vi "Test_sqlite3CreateDatabaseAndATableWorks_NoError.vi"(8 "error in (no error)":errorcluster, 11 "TestCase in":refnum<class "Test sqlite3.lvclass">) -> (0 "error out":errorcluster, 3 "TestCase out":refnum<class "Test sqlite3.lvclass">)   [LabVIEW 2020, in "Test sqlite3.lvclass"]
uses:
  Test sqlite3.lvclass
  <vilib>/Utility/sysdir.llb/System Directory Type.ctl
  externals/sqlite3/Source/sqlite3.lvclass/sqlite3.ctl
  45a547b6-e4c0-49d6-ab78-a1d3563bf804.vi
  <vilib>/Utility/error.llb/Error Cluster From Error Code.vi
  externals/sqlite3/Source/sqlite3.lvclass
  <vilib>/addons/_JKI Toolkits/VI Tester/TestCase.llb/TestCase.lvclass
  externals/database-interface/IDatabase/IDatabase/IDatabase.lvclass
  C:/Program Files/National Instruments/LabVIEW 2020/vi.lib/addons/_JKI Toolkits/VI Tester/TestCase.llb/TestCase.lvclass
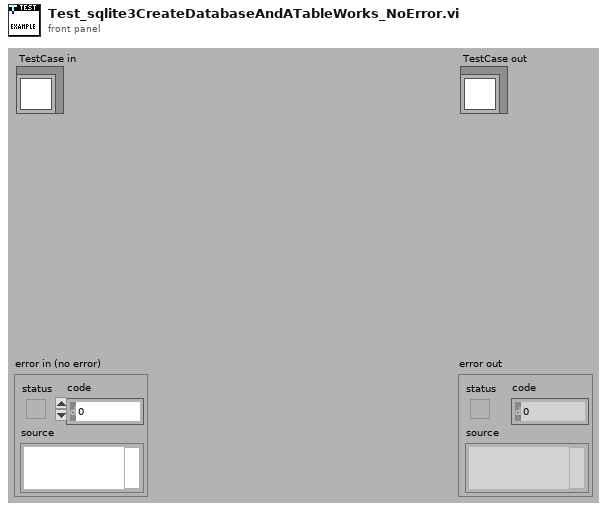
[diagram p1: front panel]
types:
  T1 = typedef "System Directory Type.ctl" = i32
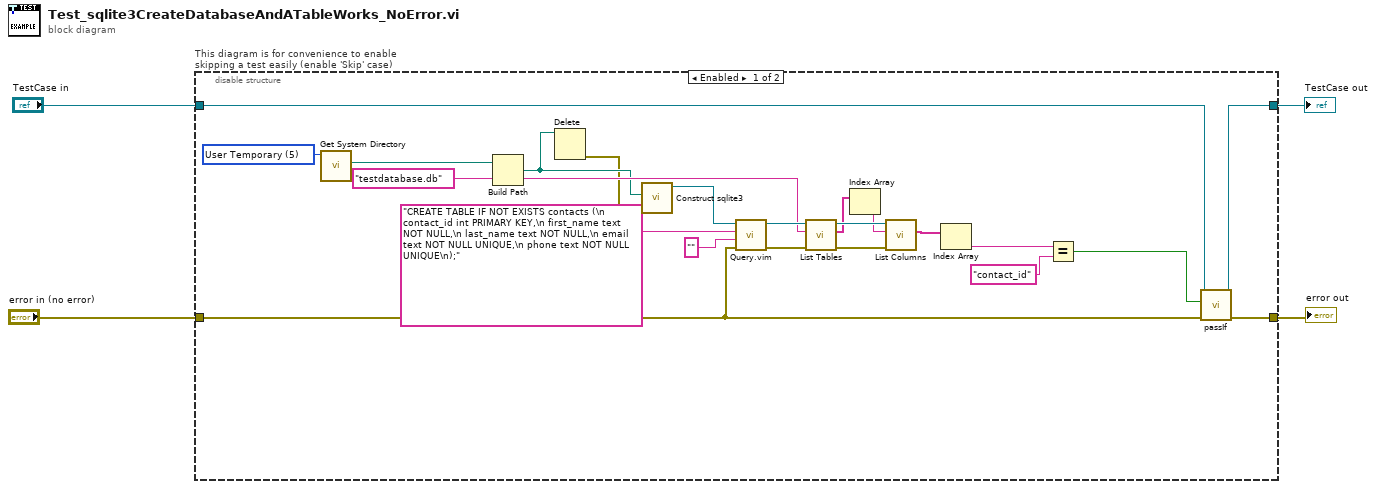
[diagram p0: block diagram]
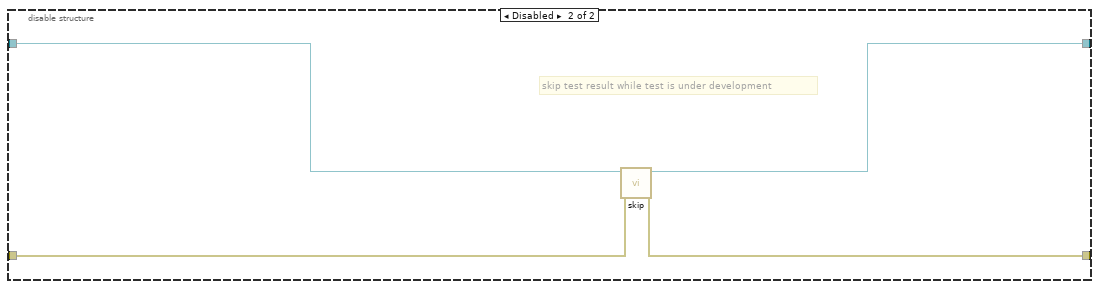
[diagram p2: hidden frame]
diagram:
  n1 = disable-structure "This diagram is for convenience to enable skipping a test easily (enable 'Skip' case)" shown="Enabled" {
    disable-tunnel: "TestCase in" -> [w24 w30]
    disable-tunnel: [w26 w28] -> w1
    disable-tunnel: [w25 w29] -> w3
    disable-tunnel: "error in (no error)" -> [w14 w27]
    frame Enabled {
      w20 = T1 5 items=["User Home"=0, "User Desktop"=1, "User Documents"=2, "User Application Data"=3, "User Preferences"=4, "User Temporary"=5, "Public Documents"=6, "Public Application Data"=7, "Public Preferences"=8, "Public Cache"=13, "System Core Libraries"=9, "System Installed Libraries"=10, "Application Files"=11, "Boot Volume Root"=12] ("system directory type")
      w13 = "testdatabase.db" ("name or relative path")
      n2 = call <vilib>:"Get System Directory.vi"("system directory type"=w20) -> ("system directory"=w19:path)  [unwired: 10 in]
      n3 = Build Path(base path=w19, name or relative path=w13) -> (appended path=w6:path)
      n4 = Delete(path (use dialog)=w6) -> (error out=w5:errorcluster)  [unwired: 4 in, 2 out]
      n5 = call "Construct sqlite3.vi"("error in (no error)"=w5, "DatabaseFilePath"=w6) -> ("sqlite3 out"=w21:refnum<class "sqlite3.lvclass">)  [unwired: 8 in, 1 out]
      n6 = call "Query.vim"("error in (no error)"=w14, "Type and Default"="" ("y"), "Query string"="CREATE TABLE IF NOT EXISTS contacts (\n contact_id int PRIMARY KEY,\n first_name text NOT NULL,\n last_name text NOT NULL,\n email text NOT NULL UNIQUE,\n phone text NOT NULL UNIQUE\n);", "IDatabase in"=w21) -> ("error out"=w16:errorcluster, "IDatabase out"=w18:refnum<class "sqlite3.lvclass">)  [unwired: 5 in, 1 out]
      n7 = call-dynamic "List Tables.vi"("error in (no error)"=w16, "Database in"=w13, "sqlite in"=w18) -> ("error out"=w15:errorcluster, "Tables out"=w12:string[], "sqlite out"=w17:refnum<class "sqlite3.lvclass">)  [unwired: 6 in]
      n8 = Index Array(array=w12) -> (element=w11:string)  [unwired: 1 in]
      n9 = call-dynamic "List Columns.vi"("error in (no error)"=w15, "Table in"=w11, "sqlite in"=w17) -> ("columns out"=w10:string[])  [unwired: 5 in, 3 out]
      n10 = Index Array(array=w10) -> (element=w9:string)  [unwired: 1 in]
      n11 = Equal?(x=w9, y="contact_id") -> (x = y?=w7:bool)
      n12 = call-dynamic "passIf.vi"("error in (no error)"=w14, "pass"=w7, "TestCase in"=w24) -> ("error out"=w25:errorcluster, "TestCase out"=w26:refnum<class "Test sqlite3.lvclass">)  [unwired: 7 in]
    }
    frame Disabled {
      # "skip test result while test is under development"
      n13 = call <vilib>:"skip.vi"("error in (no error)"=w27, "TestCase in"=w30) -> ("error out"=w29:errorcluster, "TestCase out"=w28:refnum<class "Test sqlite3.lvclass">)  [unwired: 8 in]
    }
  }
  "error out" <- w3
  "TestCase out" <- w1
